vi "Create New Palette.vi"() -> ()   [LabVIEW 2019]
doc: "This example generates a new subpalette in the User Libraries palette. Run this example before running any of the other Palette Editing API examples."
uses:
  <vilib>/Palette API/Palette Menu/Public Type Define/Palette type.ctl
  <vilib>/Palette API/Palette Menu/Public Type Define/Palette Data.ctl
  <vilib>/Palette API/Palette Menu/Public Type Define/View Format.ctl
  <vilib>/Palette API/Palette Menu/Public Type Define/Items.ctl
  <vilib>/Palette API/Palette Menu/Public Type Define/Item.ctl
  <vilib>/Palette API/Palette Menu/Public Type Define/Help Info.ctl
  <vilib>/Palette API/Palette Menu/Public Type Define/Synchronize Info.ctl
  <vilib>/Palette API/Palette Menu/Palette Menu.lvlib
panel:
  in  "palette description":string="Use the Palette API VIs\nto get/set .mnu file information."
  in  "display name":string="Palette API"
  # "Overview: Demonstrates the use of the Palette Editing VIs to create a new palette.\nInstructions:\nRun the VI. You will now have a new Functions > User Libraries > Palette API subpalette. See the block diagram for more information.\n\nNote: Several other Palette Editing API examples require that this example be run first. Once you have run all the examples and no longer need the sample subpalette, delete the following file and restart LabVIEW: [LabVIEW]\\user.lib\\PaletteAPI.mnu"
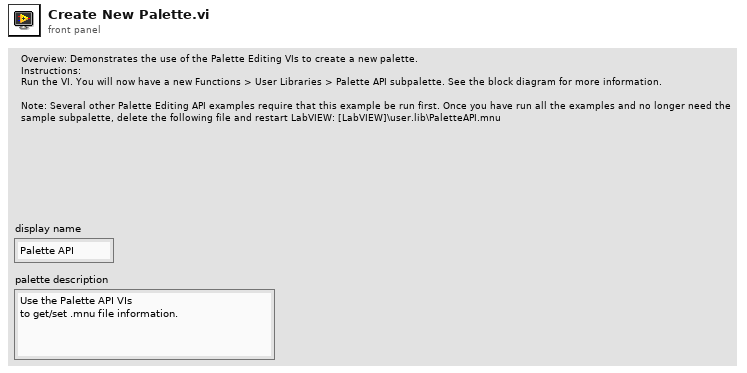
[diagram p1: front panel]
types:
  T1 = typedef "Palette Menu.lvlib/Palette Data.ctl" = cluster{"display name":string, "view format":T2, "palette width":i16, "items":T3, "256 color icon":picture, "B&W color icon":picture, "help information":T5, "palette description":string, "synchronize information":T6}
  T2 = typedef "Palette Menu.lvlib/View Format.ctl" = u16
  T3 = typedef "Palette Menu.lvlib/Items.ctl" = T4[]
  T4 = typedef "Palette Menu.lvlib/Item.ctl" = cluster{"item path":path, "library path":path, "use default lvlib palette":bool, "short name":string, "place VI contents":bool, "hide synchronized item":bool, "reserve spot for synch item":bool, "configure when placing VI contents":bool}
  T5 = typedef "Palette Menu.lvlib/Help Info.ctl" = cluster{"help tag":string, "help file path ":path}
  T6 = typedef "Palette Menu.lvlib/Synchronize Info.ctl" = cluster{"synchronize with directory":bool, "synchronize directory path":path}
  T7 = typedef "Palette Menu.lvlib/Palette type.ctl" = i32
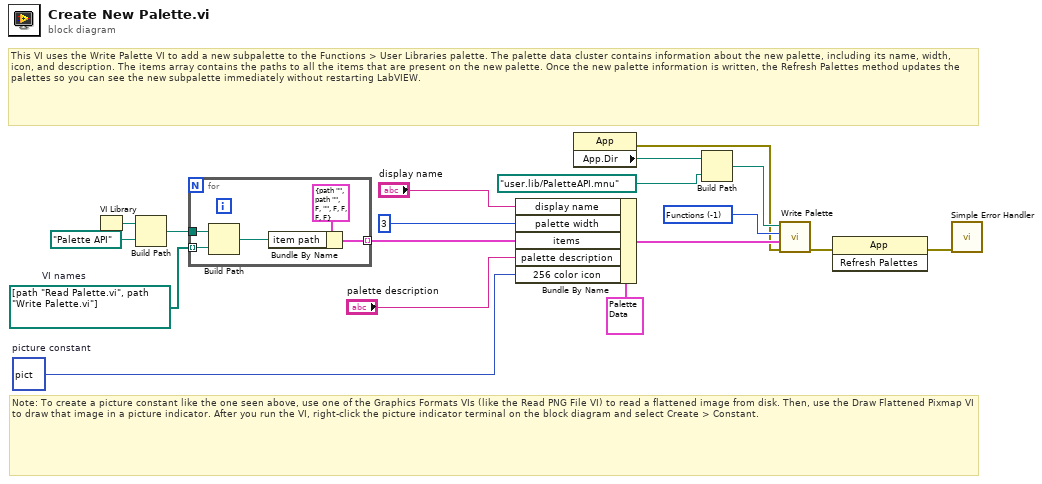
[diagram p0: block diagram]
diagram:
  w7 = T7 -1 items=["Functions"=-1, "Controls"=-2] ("palette type")
  w8 = path[] [path "Read Palette.vi", path "Write Palette.vi"]  # VI names
  w1 = picture bytes[3232]  # picture constant
  # "Note: To create a picture constant like the one seen above, use one of the Graphics Formats VIs (like the Read PNG File VI) to read a flattened image from disk. Then, use the Draw Flattened Pixmap VI to draw that image in a picture indicator. After you run the VI, right-click the picture indicator terminal on the block diagram and select Create > Constant."
  # "This VI uses the Write Palette VI to add a new subpalette to the Functions > User Libraries palette. The palette data cluster contains information about the new palette, including its name, width, icon, and description. The items array contains the paths to all the items that are present on the new palette. Once the new palette information is written, the Refresh Palettes method updates the palettes so you can see the new subpalette immediately without restarting LabVIEW."
  n1 = VI Library() -> (path=w14:path)
  n2 = Build Path(base path=w14, name or relative path=path "Palette API") -> (appended path=w12:path)
  n3 = for {
    tunnel: w8 -> [w21] mode=indexing
    tunnel: w12 -> [w20]
    tunnel: [w23] -> w15 mode=indexing
    n4 = Build Path(base path=w20, name or relative path=w21) -> (appended path=w19:path)
    n5 = Bundle By Name(cluster=T4 {"item path"=path "", "library path"=path "", "use default lvlib palette"=FALSE, "short name"="", "place VI contents"=FALSE, "hide synchronized item"=FALSE, "reserve spot for synch item"=FALSE, "configure when placing VI contents"=FALSE} ("Items"), "item path"=w19) -> (w23:T4)
  }
  n6 = Bundle By Name(cluster=T1 {"display name"="", "view format"=0, "palette width"=4, "items"=[], "256 color icon"=bytes[0], "B&W color icon"=bytes[0], "help information"={"help tag"="", "help file path "=path ""}, "palette description"="", "synchronize information"={"synchronize with directory"=FALSE, "synchronize directory path"=path ""}} ("Palette  Data"), "display name"="display name", "palette width"=i16 3, "items"=w15, "palette description"="palette description", "256 color icon"=w1) -> (w18:T1)
  n7 = property class="App"() -> (error out=w3:errorcluster, "App.Dir"=w6:path)  [unwired: 2 in, 1 out]
  n8 = Build Path(base path=w6, name or relative path=path "user.lib/PaletteAPI.mnu") -> (appended path=w16:path)
  n9 = call <vilib>:"Write Palette.vi"("error in (no error)"=w3, "palette data"=w18, "palette type"=w7, "palette path"=w16) -> ("error out"=w11:errorcluster)  [unwired: 1 in, 6 out]
  n10 = invoke class="App" method="Refresh Palettes"(error in=w11) -> (error out=w10:errorcluster)  [unwired: 2 in, 2 out]
  n11 = call <vilib>:"Simple Error Handler.vi"("error in (no error)"=w10) -> ()  [unwired: 1 in, 8 out]
